vi "01_FRA_Data_converter.vi"() -> ()   [LabVIEW 2013]
uses:
  subVIs/Data_conv_UI.ctl
  <vilib>/Utility/file.llb/Read From Spreadsheet File (string).vi
panel:
  in  "Scan file for units":bool
  in  "Run conversion":bool
  out "Volts file path":path caption="selected path"
  out "Source file path":path caption="selected path"
  in  "Stop VI":bool
  in  "App-specific conv.":bool
  in  "File selection":bool
  out "Processing row":string
  in  "format string":string="%f"
  out "Processing row #":i32
  out "Header":string
  # "FRA Unit LabVIEW data converter"
  # "Configuration"
  # "Converter to volts (*_volts.csv)"
  # "App-specific conversion settings:"
  # "Volts to application-specific"
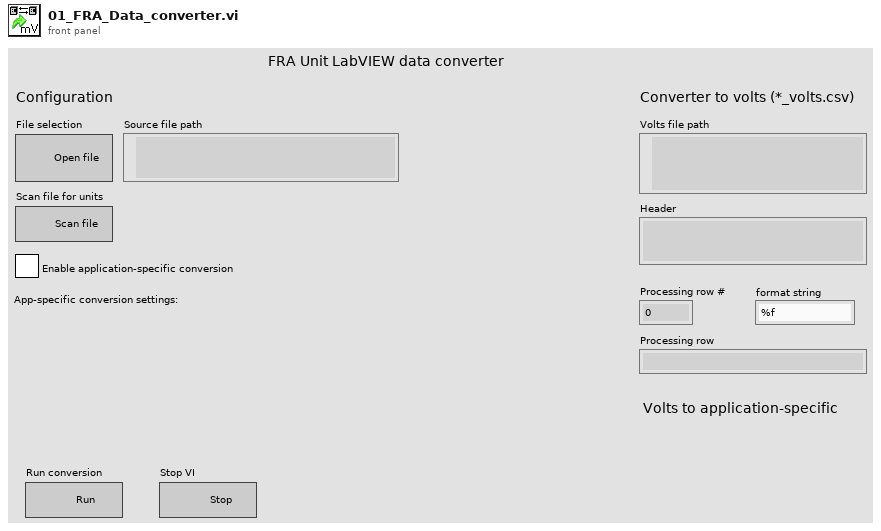
[diagram p1: front panel]
types:
  T1 = typedef "Data_conv_UI.ctl" = enum16{"Stop", "OpenFile", "ScanFIle", "ConvToVolts", "ConvToApp"}
  T2 = enum16{"open", "replace", "create", "open or create", "replace or create", "replace or create with confirmation"}
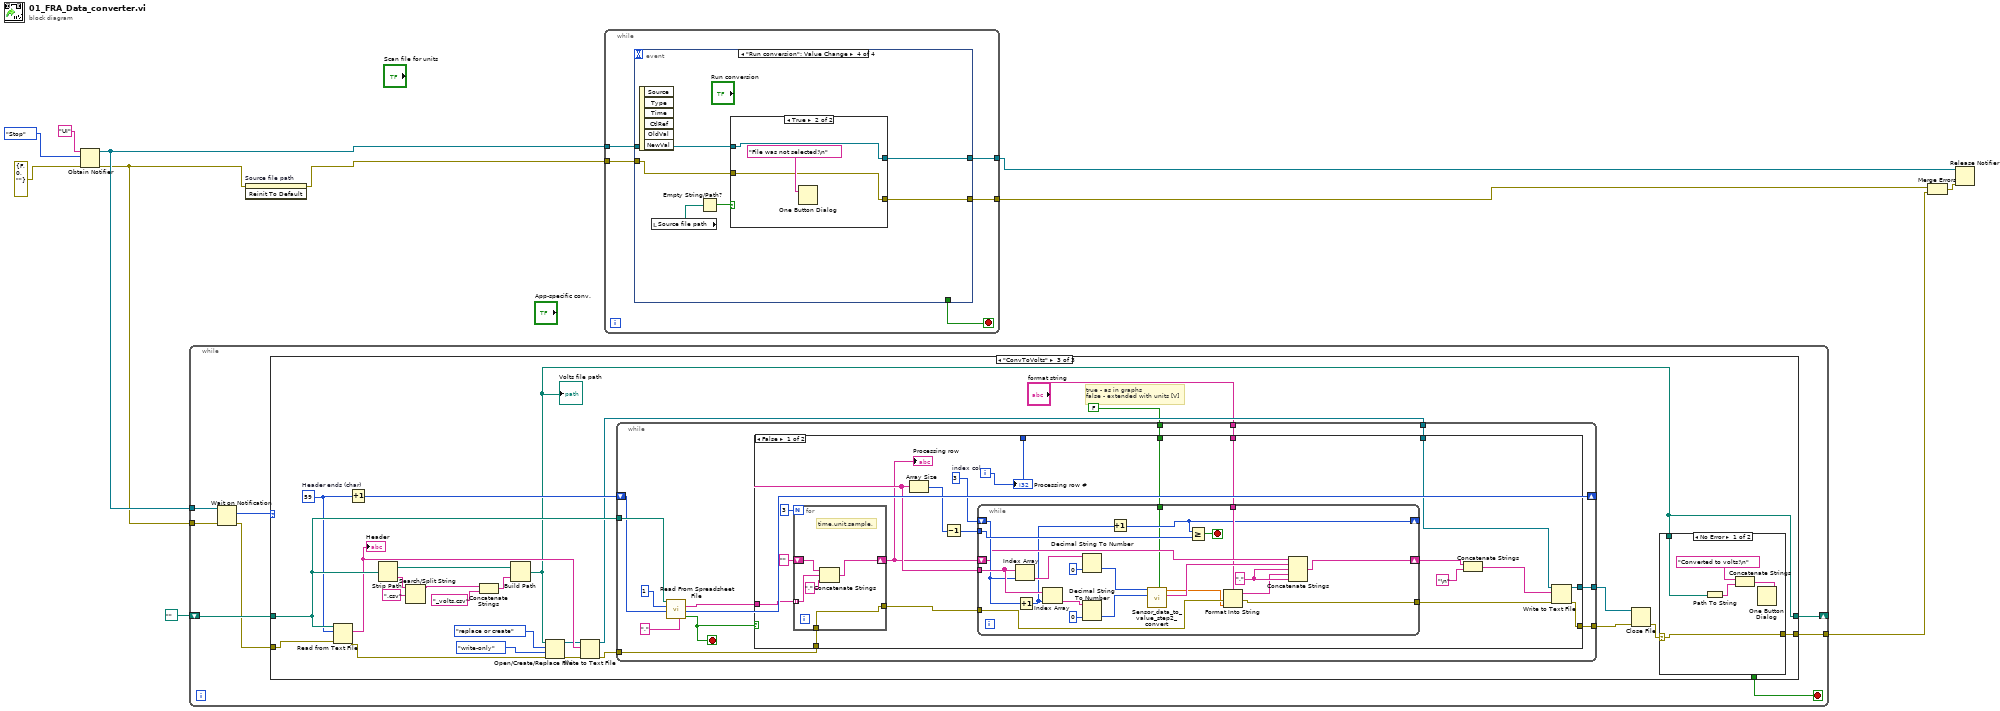
[diagram p0: block diagram]
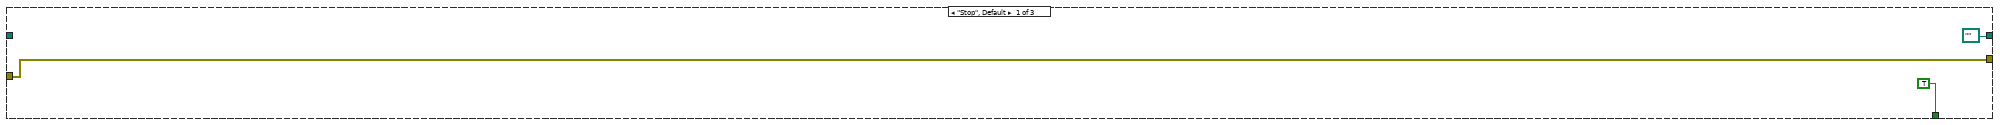
[diagram p2: hidden frame]
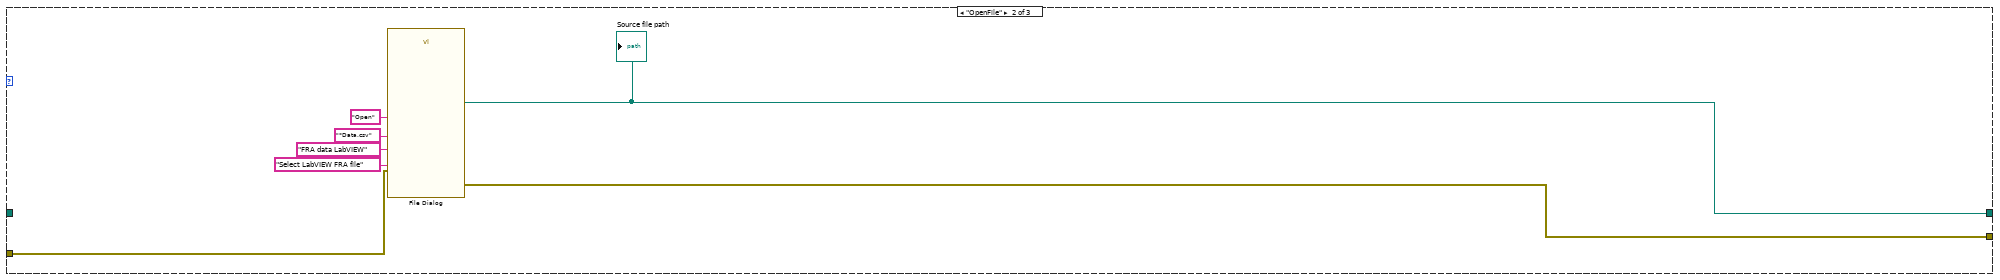
[diagram p3: hidden frame]
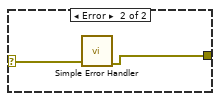
[diagram p4: hidden frame]
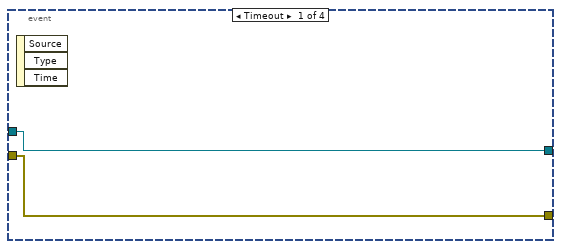
[diagram p6: hidden frame]
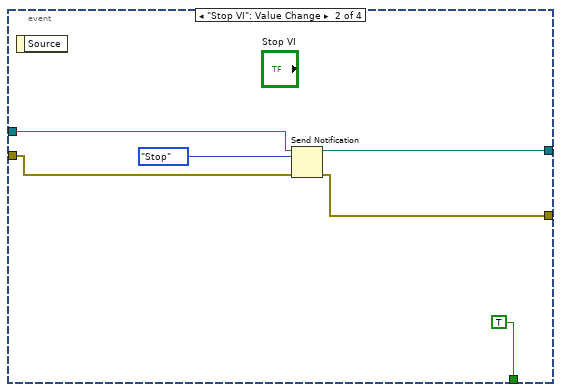
[diagram p7: hidden frame]
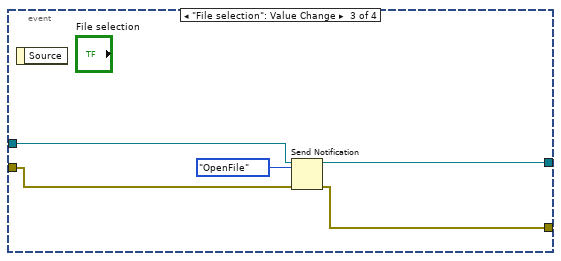
[diagram p8: hidden frame]
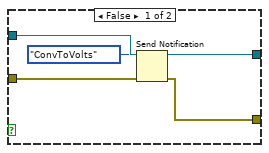
[diagram p9: hidden frame]
diagram:
  n1 = Obtain Notifier(name (unnamed)="UI", notification data type=Data_conv_UI."Stop" ("Enum"), error in (no error)=errorcluster {"status"=FALSE, "code"=0, "source"=""} ("error constant")) -> (notifier out=w7:refnum<notifier>, error out=w2:errorcluster)  [unwired: 1 in, 1 out]
  n2 = while {
    shift-right: [w12] -> _
    shift-left: path "" ("selected path") -> [w19]
    tunnel: w7 -> [w18]
    tunnel: w2 -> [w17]
    tunnel: [w13] -> w4
    stop <- w14 stop-if-true
    n3 = Wait on Notification(notifier=w18, error in (no error)=w17) -> (notification=w16:T1, error out=w15:errorcluster)  [unwired: 2 in, 2 out]
    n4 = case shown="\"ConvToVolts\"" w16 {
      tunnel: w19 -> [_ _ w54]
      tunnel: w15 -> [w21 w25 w33]
      tunnel: [TRUE _ _] -> w14
      tunnel: [w21 w24 w30] -> w13
      tunnel: [path "" ("selected path") w23 w31] -> w12
      frame "Stop", Default {
      }
      frame "OpenFile" {
        n5 = call "File Dialog"("prompt"="Select LabVIEW FRA file", "button label"="Open", "error in"=w25, "pattern (all files)"="*Data.csv", "pattern label"="FRA data LabVIEW") -> ("selected path"=w23:path, "error out"=w24:errorcluster)  [unwired: 7 in, 2 out]
        "Source file path" <- w23
      }
      frame "ConvToVolts" {
        w41 = 59  # Header ends (char)
        # "true - as in graphs\nfalse - extended with units [V]"
        n6 = Read from Text File(file (use dialog)=w54, count=w41, error in=w33) -> (text=w44:string, error out=w39:errorcluster)  [unwired: 1 in, 2 out]
        "Header" <- w44
        n7 = Increment(x=w41) -> (x+1=w40:i32)
        n8 = Strip Path(path=w54) -> (stripped path=w53:path, name=w48:string)
        n9 = Search/Split String(string=w48, search string/char (-)=".csv") -> (substring before match=w47:string)  [unwired: 1 in, 2 out]
        n10 = Concatenate Strings(w47, "_volts.csv" ("string")) -> (w52:string)
        n11 = Build Path(base path=w53, name or relative path=w52) -> (appended path=w31:path)
        "Volts file path" <- w31
        n12 = Open/Create/Replace File(file path (use dialog)=w31, error in=w39, operation (0:open)=T2."replace or create", access (0:read/write)=enum16{"read/write", "read-only", "write-only"}."write-only") -> (refnum out=w43:refnum<file>, error out=w45:errorcluster)  [unwired: 2 in, 1 out]
        n13 = Write to Text File(file (use dialog)=w43, text=w44, error in=w45) -> (refnum out=w38:refnum<file>, error out=w42:errorcluster)  [unwired: 1 in, 1 out]
        n14 = while {
          tunnel: w42 -> [w69]
          tunnel: w54 -> [w72]
          shift-right: [w70] -> _
          shift-left: w40 -> [w71]
          tunnel: w38 -> [w66]
          tunnel: [w65] -> w32
          tunnel: "format string" -> [w67]
          tunnel: [w64] -> w36
          tunnel: FALSE -> [w62]
          i -> [w75]
          stop <- w63 stop-if-true
          n15 = call-poly <vilib>:"Read From Spreadsheet File.vi"("delimiter (\\t)"="," ("delimiter (\\t)"), "start of read offset (chars.:0)"=w71, "number of rows (all:-1)"=1, "file path (dialog if empty)"=w72) -> ("EOF?"=w63:bool, "mark after read (chars.)"=w70:i32, "first row"=w68:string[])  [unwired: 3 in, 2 out]
          n16 = case shown="False" w63 {
            tunnel: w75 -> [w94 _]
            tunnel: w69 -> [w92 w123]
            tunnel: w68 -> [w87 _]
            tunnel: w67 -> [w86 _]
            tunnel: w66 -> [w84 w122]
            tunnel: [w83 w122] -> w65
            tunnel: [w82 w123] -> w64
            tunnel: w62 -> [w76 _]
            frame False {
              w91 = 3  # index col
              n17 = for {
                N: 3 -> [_]
                tunnel: w87 -> [w121] mode=indexing
                tunnel: w92 -> [w119]
                tunnel: [w119] -> w90
                shift-right: [w117] -> w77
                shift-left: "" -> [w118]
                # "time,unit,sample,"
                n18 = Concatenate Strings(w118, w121, "," ("string")) -> (w117:string)
              }
              "Processing row" <- w77
              n19 = Array Size(array=w87) -> (size(s)=w89:i32)
              n20 = Decrement(x=w89) -> (x-1=w78:i32)
              n21 = while {
                tunnel: w90 -> [w102]
                shift-right: [w97] -> _
                shift-left: w91 -> [w113]
                tunnel: w78 -> [w116]
                shift-right: [w107] -> w81
                shift-left: w77 -> [w106]
                tunnel: w87 -> [w114]
                tunnel: w86 -> [w100]
                tunnel: [w99] -> w85
                tunnel: w76 -> [w95]
                stop <- w115 stop-if-true
                w104 = "," ("string")
                n22 = Index Array(array=w114, index=w113) -> (element=w112:string)
                n23 = Increment(x=w113) -> (x+1=w98:i32)
                n24 = Index Array(array=w114, index=w98) -> (element=w111:string)
                n25 = Decimal String To Number(string=w112, default (0L)=u8 0 ("default (0 I32)")) -> (number=w108:u8)  [unwired: 1 in, 1 out]
                n26 = Decimal String To Number(string=w111, default (0L)=0 ("default (0 I32)")) -> (number=w96:i32)  [unwired: 1 in, 1 out]
                n27 = Increment(x=w98) -> (x+1=w97:i32)
                n28 = call "Sensor_data_to_value_step2_convert.vi"("Graph format (T)"=w95, "Sensor data resolved sign"=w96, "Sensor type"=w108) -> ("Signal legend"=w105:string, "Value ouptut"=w101:dbl)  [unwired: 7 in]
                n29 = Greater Or Equal?(x=w97, y=w116) -> (x >= y?=w115:bool)
                n30 = Format Into String(format string=w100, error in=w102, w101) -> (resulting string=w103:string, error out=w99:errorcluster)  [unwired: 1 in]
                n31 = Concatenate Strings(w106, w105, w104, w103, w104) -> (w107:string)
              }
              n32 = Concatenate Strings(w81, "\n" ("string")) -> (w79:string)
              n33 = Write to Text File(file (use dialog)=w84, text=w79, error in=w85) -> (refnum out=w83:refnum<file>, error out=w82:errorcluster)  [unwired: 1 in, 1 out]
              "Processing row #" <- w94
            }
            frame True {
            }
          }
        }
        n34 = Close File(refnum=w32, error in=w36) -> (error out=w35:errorcluster)  [unwired: 1 out]
        n35 = case shown="No Error" w35 {
          selector: w35 -> [w55 w61]
          tunnel: w31 -> [w56 _]
          tunnel: [w55 w60] -> w30
          frame No Error {
            n36 = Path To String(path=w56) -> (string=w57:string)
            n37 = Concatenate Strings("Converted to volts!\n" ("message"), w57) -> (w58:string)
            n38 = One Button Dialog(message=w58) -> ()  [unwired: 1 in, 1 out]
          }
          frame Error {
            n39 = call <vilib>:"Simple Error Handler.vi"("error in (no error)"=w61) -> ("error out"=w60:errorcluster)  [unwired: 4 in, 4 out]
          }
        }
      }
    }
  }
  n40 = invoke on="Source file path" class="Path" method="Reinit To Default"(error in=w2) -> (error out=w1:errorcluster)  [unwired: 2 in, 2 out]
  n41 = while {
    tunnel: w7 -> [w127]
    tunnel: w1 -> [w128]
    tunnel: [w126] -> w8
    tunnel: [w124] -> w3
    stop <- w125 stop-if-true
    n42 = event shown="[3] \"Run conversion\": Value Change" {
      selector: _ -> [_ _ _ _]
      dyn-events: _ -> [_ _ _ _]
      timeout: _ -> [_ _ _ _]
      tunnel: w128 -> [w129 w135 w140 w146]
      tunnel: w127 -> [w130 w136 w141 w147]
      tunnel: [w130 w133 w139 w145] -> w126
      tunnel: [_ TRUE _ _] -> w125
      tunnel: [w129 w131 w138 w144] -> w124
      event Timeout {
        n43 = event-data() -> ()  [unwired: 1 in, 3 out]
      }
      event "Stop VI": Value Change {
        n44 = event-data() -> ()  [unwired: 1 in, 1 out]
        n45 = Send Notification(notification=Data_conv_UI."Stop" ("Enum"), notifier=w136, error in (no error)=w135) -> (notifier out=w133:refnum<notifier>, error out=w131:errorcluster)
      }
      event "File selection": Value Change {
        n46 = event-data() -> ()  [unwired: 1 in, 1 out]
        n47 = Send Notification(notification=Data_conv_UI."OpenFile" ("Enum"), notifier=w141, error in (no error)=w140) -> (notifier out=w139:refnum<notifier>, error out=w138:errorcluster)
      }
      event "Run conversion": Value Change {
        n48 = event-data() -> ()  [unwired: 1 in, 6 out]
        n49 = local read "Source file path"() -> (w142:path)
        n50 = Empty String/Path?(string/path=w142) -> (empty?=w143:bool)
        n51 = case shown="True" w143 {
          tunnel: w147 -> [w152 w154]
          tunnel: w146 -> [w151 w153]
          tunnel: [w149 w154] -> w145
          tunnel: [w148 w153] -> w144
          frame False {
            n52 = Send Notification(notification=Data_conv_UI."ConvToVolts" ("Enum"), notifier=w152, error in (no error)=w151) -> (notifier out=w149:refnum<notifier>, error out=w148:errorcluster)
          }
          frame True {
            n53 = One Button Dialog(message="File was not selected!\n") -> ()  [unwired: 1 in, 1 out]
          }
        }
      }
    }
  }
  n54 = Merge Errors(w3, w4) -> (w5:errorcluster)
  n55 = Release Notifier(notifier=w8, error in (no error)=w5) -> ()  [unwired: 1 in, 3 out]
